vi "write data.vi"() -> ()   [LabVIEW 2020]
uses:
  <vilib>/Utility/file.llb/Read Delimited Spreadsheet (DBL).vi
  <vilib>/Utility/file.llb/Write Delimited Spreadsheet (DBL).vi
panel:
  out "Array":dbl[][](array[numeric])
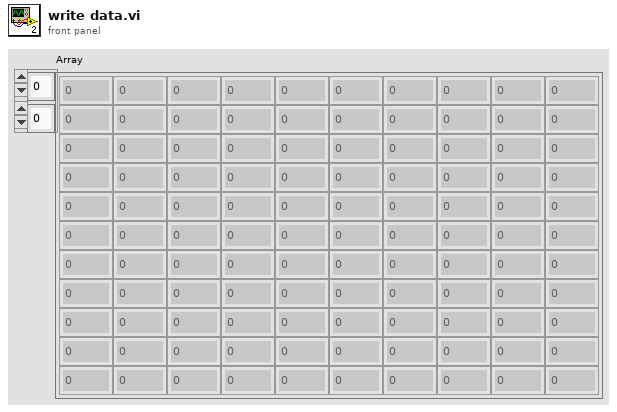
[diagram p1: front panel]
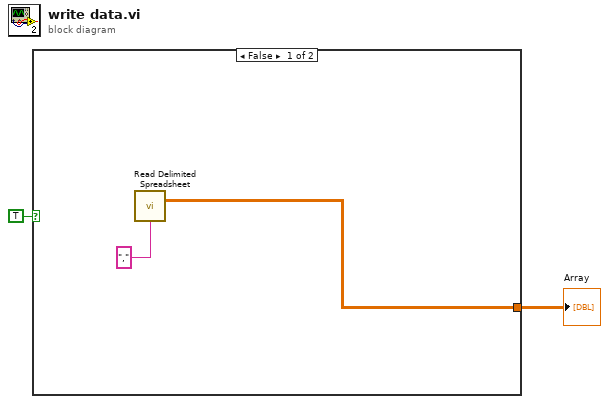
[diagram p0: block diagram]
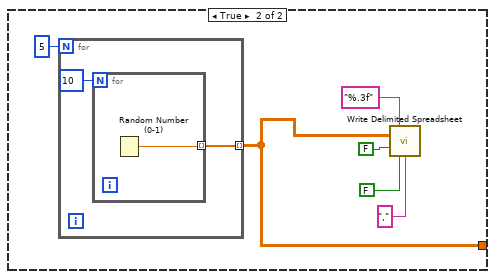
[diagram p2: hidden frame]
diagram:
  n1 = case shown="False" TRUE {
    tunnel: [w4 w9] -> w2
    frame False {
      n2 = call-poly <vilib>:"Read Delimited Spreadsheet.vi"("delimiter (\\t)"="," ("delimiter (\\t)")) -> ("all rows"=w4:dbl[][])  [unwired: 9 in, 5 out]
    }
    frame True {
      n3 = for {
        N: 5 -> [_]
        tunnel: [w12] -> w9 mode=indexing
        n4 = for {
          N: 10 -> [_]
          tunnel: [w13] -> w12 mode=indexing
          n5 = Random Number (0-1)() -> (number: 0 to 1=w13:dbl)
        }
      }
      n6 = call-poly <vilib>:"Write Delimited Spreadsheet.vi"("format (%.3f)"="%.3f", "2D data"=w9, "append to file? (new file:F)"=FALSE, "transpose? (no:F)"=FALSE, "delimiter (\\t)"="," ("delimiter (\\t)")) -> ()  [unwired: 9 in, 2 out]
    }
  }
  "Array" <- w2
